vi "Store Configuration Parameters.vi"(8 "error in (no error)":errorcluster, 10 "refnum":T1, 11 "DAQ Configuration in":refnum<class "DAQ Configuration.lvclass">) -> (0 "error out":errorcluster, 2 "refnum out":T1, 3 "DAQ Configuration out":refnum<class "DAQ Configuration.lvclass">)   [LabVIEW 2026, in "Hardware.lvlib" / "DAQ Configuration.lvclass"]
uses:
  DAQ Configuration.lvclass
  <vilib>/Utility/config.llb/Config Data RefNum.ctl
  DAQ Configuration.lvclass/DAQ Configuration.ctl
  framework/Hardware/HW with output config.lvclass
  <vilib>/Utility/config.llb/NI_LVConfig.lvlib
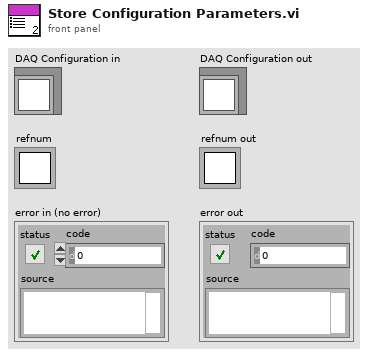
[diagram p1: front panel]
types:
  T1 = typedef "NI_LVConfig.lvlib/Config Data RefNum.ctl" = refnum<k1>
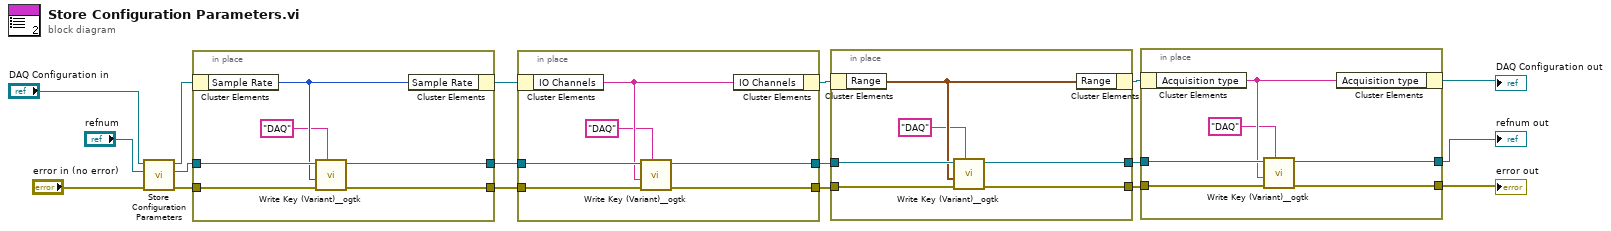
[diagram p0: block diagram]
diagram:
  n1 = call-parent "Store Configuration Parameters.vi"("error in (no error)"="error in (no error)", "refnum"="refnum", "HW with output config in"="DAQ Configuration in") -> ("error out"=w13:errorcluster, "refnum out"=w14:T1, "HW with output config out"=w15:refnum<class "DAQ Configuration.lvclass">)  [unwired: 6 in]
  n2 = in-place "In Place Element Structure" {
    in-place-border: w14 -> [w24]
    in-place-border: w13 -> [w23]
    in-place-border: [w20] -> w10
    in-place-border: [w19] -> w11
    n3 = in-place-cluster #1(w15) -> ("Sample Rate"=w22:i32)
    n4 = call <userlib>:"Write Key (Variant)__ogtk.vi"("section"="DAQ", "error in (no error)"=w23, "key-value"=w22, "refnum"=w24) -> ("error out"=w20:errorcluster, "refnum out"=w19:T1)  [unwired: 6 in]
    n5 = in-place-cluster #1("Sample Rate"=w22) -> (w12:refnum<class "DAQ Configuration.lvclass">)
  }
  n6 = in-place "In Place Element Structure" {
    in-place-border: w11 -> [w30]
    in-place-border: w10 -> [w29]
    in-place-border: [w26] -> w8
    in-place-border: [w25] -> w9
    n7 = in-place-cluster #2(w12) -> ("IO Channels"=w28:string)
    n8 = call <userlib>:"Write Key (Variant)__ogtk.vi"("section"="DAQ", "error in (no error)"=w29, "key-value"=w28, "refnum"=w30) -> ("error out"=w26:errorcluster, "refnum out"=w25:T1)  [unwired: 6 in]
    n9 = in-place-cluster #2("IO Channels"=w28) -> (w7:refnum<class "DAQ Configuration.lvclass">)
  }
  n10 = in-place "In Place Element Structure" {
    in-place-border: w9 -> [w36]
    in-place-border: w8 -> [w35]
    in-place-border: [w32] -> w5
    in-place-border: [w31] -> w6
    n11 = in-place-cluster #3(w7) -> ("Range"=w34:cluster{"Ranve (min)":dbl, "Range Max":dbl})
    n12 = call <userlib>:"Write Key (Variant)__ogtk.vi"("section"="DAQ", "error in (no error)"=w35, "key-value"=w34, "refnum"=w36) -> ("error out"=w32:errorcluster, "refnum out"=w31:T1)  [unwired: 6 in]
    n13 = in-place-cluster #3("Range"=w34) -> (w4:refnum<class "DAQ Configuration.lvclass">)
  }
  n14 = in-place "In Place Element Structure" {
    in-place-border: w6 -> [w42]
    in-place-border: w5 -> [w41]
    in-place-border: [w38] -> w3
    in-place-border: [w37] -> w2
    n15 = in-place-cluster #4(w4) -> ("Acquisition type"=w40:string)
    n16 = call <userlib>:"Write Key (Variant)__ogtk.vi"("section"="DAQ", "error in (no error)"=w41, "key-value"=w40, "refnum"=w42) -> ("error out"=w38:errorcluster, "refnum out"=w37:T1)  [unwired: 6 in]
    n17 = in-place-cluster #4("Acquisition type"=w40) -> (→"DAQ Configuration out":refnum<class "DAQ Configuration.lvclass">)
  }
  "error out" <- w3
  "refnum out" <- w2
